vi "Actor Core.vi"(8 "error in":errorcluster, 11 "Shaker Controller in":refnum<class "Shaker Controller.lvclass">) -> (0 "error out":errorcluster, 3 "Actor out":refnum<class "Actor.lvclass">)   [LabVIEW 2020, in "Shaker Controller.lvlib" / "Shaker Controller.lvclass"]
doc: "(<B>Filename</B>: Actor Framework.lvlib:Actor.lvclass:Actor Core.vi)\n\nReceives messages to the actor, reacts to them, and initiates any error handling that may shut the actor down.\n\nDescendant classes may override this VI to append parallel tasks for the actor to complete while it handles messages. Overrides use the Call Parent Class Method node."
uses:
  Shaker Controller.lvclass
  C:/Program Files (x86)/National Instruments/LabVIEW 2020/vi.lib/ActorFramework/Actor/Actor.lvclass
  <vilib>/ActorFramework/Actor/Actor.lvclass
  Shaker Controller Messages/Read Shake Data Msg/Read Shake Data Msg.lvclass
  C:/Program Files (x86)/National Instruments/LabVIEW 2020/vi.lib/ActorFramework/Message/Message.lvclass
  <vilib>/ActorFramework/Actor/Actor.lvclass/Actor.ctl
  <vilib>/ActorFramework/Message Enqueuer/Message Enqueuer.lvclass/Message Enqueuer.ctl
  <vilib>/ActorFramework/Message Enqueuer/Init from Existing Queue.vi
  <vilib>/ActorFramework/Message Enqueuer/Enqueue.vi
  Shaker Controller Interface/Shaker Controller Interface Messages/Shaker Controller Initialized Msg/Shaker Controller Initialized Msg.lvclass
  <vilib>/ActorFramework/Message Priority Queue/Priority Enqueue.vi
  <vilib>/MGI/Monitored Actor/Monitored Actor/Monitored Actor/Monitored Actor.lvclass
  <vilib>/ActorFramework/Message Enqueuer/Message Enqueuer.lvclass
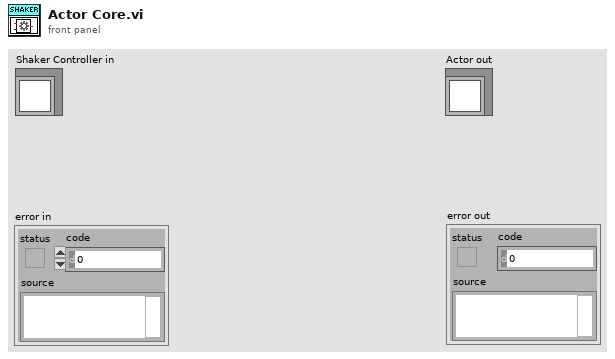
[diagram p1: front panel]
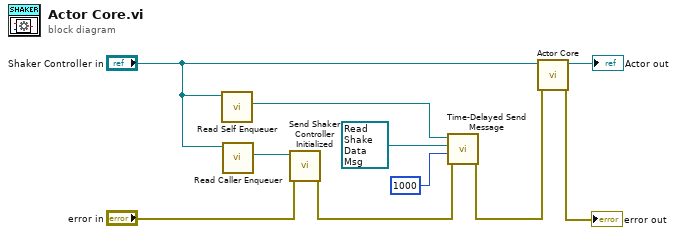
[diagram p0: block diagram]
diagram:
  n1 = call <vilib>:"Read Self Enqueuer.vi"("Actor"="Shaker Controller in") -> ("Self Enqueuer"=w6:refnum<class "Message Enqueuer.lvclass">)  [unwired: 10 in]
  n2 = call <vilib>:"Read Caller Enqueuer.vi"("Actor"="Shaker Controller in") -> ("Caller Enqueuer"=w8:refnum<class "Message Enqueuer.lvclass">)  [unwired: 10 in]
  n3 = call "Send Shaker Controller Initialized.vi"("error in (no error)"="error in", "Message Enqueuer"=w8) -> ("error out"=w3:errorcluster)  [unwired: 8 in, 1 out]
  n4 = call <vilib>:"Time-Delayed Send Message.vi"("error in (no error)"=w3, "Milliseconds To Wait"=1000, "Message"=refnum<class "Read Shake Data Msg.lvclass"> refnum ("Shaker Controller.lvlib:Read Shake Data Msg.lvclass"), "Message Enqueuer"=w6) -> ("error out"=w2:errorcluster)  [unwired: 6 in, 1 out]
  n5 = call-parent "Actor Core.vi"("error in"=w2, "Actor in"="Shaker Controller in") -> ("error out"=→"error out":errorcluster, "Actor out"=→"Actor out":refnum<class "Actor.lvclass">)  [unwired: 8 in]
